vi "destroyReferences.vi"(8 "error in (no error)":errorcluster, 11 "tcpServerCmd in":refnum<class "TcpServerCmd.lvclass">) -> (0 "error out":errorcluster, 3 "tcpServerCmd out":refnum<class "TcpServerCmd.lvclass">)   [LabVIEW 2018, in "TcpServerCmd.lvclass"]
doc: "Destroy the notifierStopServer, serverNotifier, and GenRead references."
uses:
  TcpServerCmd.lvclass
  home/pcortes/Documents/github/ts_labview_tcp_json/src/TcpServerBase/TcpServerBase.lvclass
  TcpServerBase/TcpServerBase.lvclass
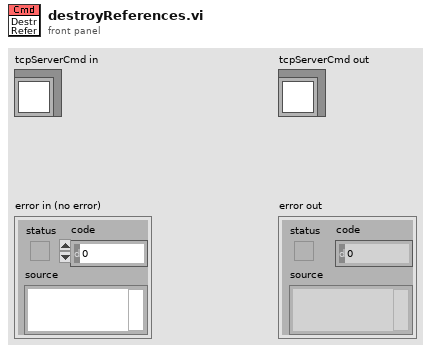
[diagram p1: front panel]
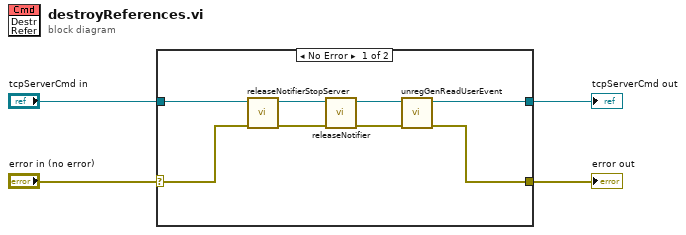
[diagram p0: block diagram]
diagram:
  n1 = case shown="No Error" "error in (no error)" {
    selector: "error in (no error)" -> [w11 w14]
    tunnel: "tcpServerCmd in" -> [w12 w13]
    tunnel: [w6 w13] -> w3
    tunnel: [w5 w14] -> w1
    frame No Error {
      n2 = call "releaseNotifierStopServer.vi"("error in (no error)"=w11, "tcpServerBase in"=w12) -> ("error out"=w9:errorcluster, "tcpServerBase out"=w10:refnum<class "TcpServerCmd.lvclass">)  [unwired: 8 in]
      n3 = call "releaseNotifier.vi"("error in (no error)"=w9, "tcpServerBase in"=w10) -> ("error out"=w7:errorcluster, "tcpServerBase out"=w8:refnum<class "TcpServerCmd.lvclass">)  [unwired: 8 in]
      n4 = call "unregGenReadUserEvent.vi"("error in (no error)"=w7, "tcpServerBase in"=w8) -> ("error out"=w5:errorcluster, "tcpServerBase out"=w6:refnum<class "TcpServerCmd.lvclass">)  [unwired: 8 in]
    }
    frame Error {
    }
  }
  "tcpServerCmd out" <- w3
  "error out" <- w1
